vi "RandomNumberMatchesInput.vi"() -> ()   [LabVIEW 2015]
panel:
  out "Time in seconds":dbl
  out "Iteration Count":i32=1432
  in  "Delay in ms":u32=10
  out "Done":bool=TRUE
  out "Generated Number":u32=120
  in  "Input Number":u32=50
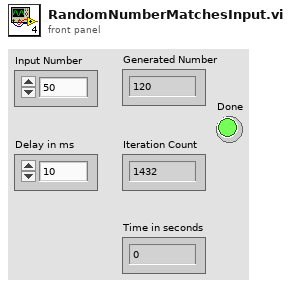
[diagram p1: front panel]
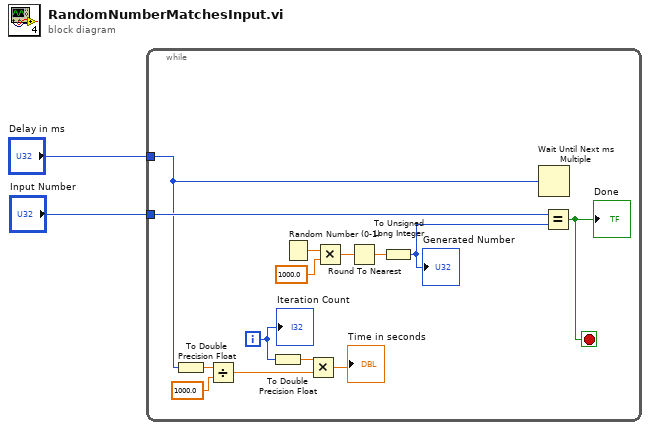
[diagram p0: block diagram]
diagram:
  n1 = while {
    tunnel: "Input Number" -> [w11]
    tunnel: "Delay in ms" -> [w4]
    i -> [w8]
    stop <- w10 stop-if-true
    n2 = To Double Precision Float(number=w4) -> (double precision float=w5:dbl)
    n3 = Divide(x=w5, y=1000.0) -> (x/y=w3:dbl)
    n4 = To Double Precision Float(number=w8) -> (double precision float=w9:dbl)
    n5 = Random Number (0-1)() -> (number: 0 to 1=w13:dbl)
    n6 = Multiply(x=w9, y=w3) -> (x*y=→"Time in seconds":dbl)
    n7 = Multiply(x=w13, y=1000.0) -> (x*y=w15:dbl)
    n8 = Round To Nearest(number=w15) -> (nearest integer value=w16:dbl)
    n9 = To Unsigned Long Integer(number=w16) -> (unsigned 32bit integer=w12:u32)
    "Generated Number" <- w12
    n10 = Wait Until Next ms Multiple(millisecond multiple=w4) -> ()  [unwired: 1 out]
    n11 = Equal?(x=w11, y=w12) -> (x = y?=w10:bool)
    "Done" <- w10
    "Iteration Count" <- w8
  }
